vi "test Set Change on Parent.vi"(8 "error in":errorcluster, 11 "TestCase in":refnum<class "Refresh.lvclass">) -> (0 "error out":errorcluster, 3 "TestCase out":refnum<class "Refresh.lvclass">)   [LabVIEW 2020, in "Refresh.lvclass"]
uses:
  Refresh.lvclass
  System Explorer/Implementation/System Explorer/Refresh/MCL Row.ctl
  System Explorer/Implementation/System Explorer/Refresh/Change Type.ctl
  System Explorer/Implementation/System Explorer/Refresh/Symbols.ctl
  Scripting/Constants.vi
  <vilib>/addons/_JKI Toolkits/VI Tester/TestCase.llb/TestCase.lvclass
  System Explorer/Implementation/System Explorer/Refresh/Refresh.lvlib
  Scripting/AIM MIL-STD-1553 Scripting.lvlib
  C:/Program Files (x86)/National Instruments/LabVIEW 2020/vi.lib/addons/_JKI Toolkits/VI Tester/TestCase.llb/TestCase.lvclass
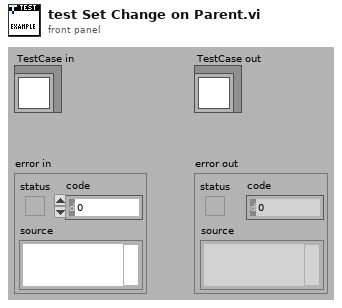
[diagram p1: front panel]
types:
  T1 = typedef "AIM MIL-STD-1553 System Explorer.lvlib/Implementation.lvlib/Refresh.lvlib/MCL Row.ctl" = cluster{"change type":T2, "item symbol":T3, "item names":string[]}
  T2 = typedef "AIM MIL-STD-1553 System Explorer.lvlib/Implementation.lvlib/Refresh.lvlib/Change Type.ctl" = enum16{"No change", "Modify", "Add", "Remove"}
  T3 = typedef "AIM MIL-STD-1553 System Explorer.lvlib/Implementation.lvlib/Refresh.lvlib/Symbols.ctl" = enum16{"Blank", "MIL-STD-1553", "Port", "Remote Terminal", "Subaddress", "Bus Controller", "Frame", "Mode Code", "Message", "Parameter", "Item"}
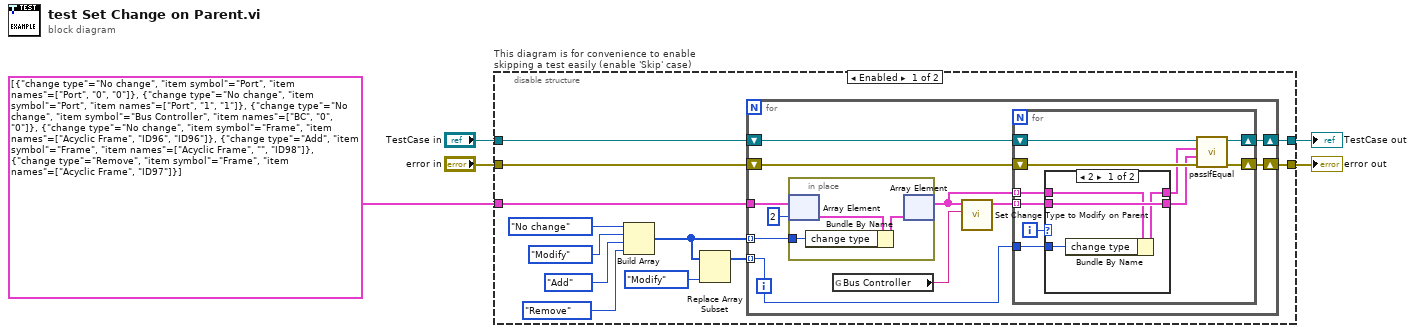
[diagram p0: block diagram]
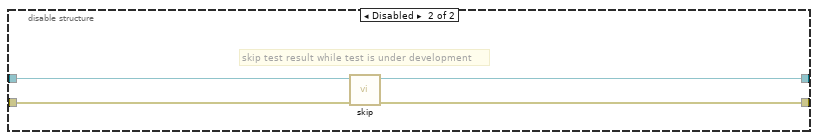
[diagram p3: hidden frame]
diagram:
  n1 = disable-structure "This diagram is for convenience to enable skipping a test easily (enable 'Skip' case)" shown="Enabled" {
    disable-tunnel: "TestCase in" -> [w17 w51]
    disable-tunnel: [w15 w49] -> w2
    disable-tunnel: [w14 w50] -> w4
    disable-tunnel: "error in" -> [w16 w48]
    disable-tunnel: T1[] [{"change type"=enum."No change", "item symbol"=enum."Port", "item names"=["Port", "0", "0"]}, {"change type"=enum."No change", "item symbol"=enum."Port", "item names"=["Port", "1", "1"]}, {"change type"=enum."No change", "item symbol"=enum."Bus Controller", "item names"=["BC", "0", "0"]}, {"change type"=enum."No change", "item symbol"=enum."Frame", "item names"=["Acyclic Frame", "ID96", "ID96"]}, {"change type"=enum."Add", "item symbol"=enum."Frame", "item names"=["Acyclic Frame", "", "ID98"]}, {"change type"=enum."Remove", "item symbol"=enum."Frame", "item names"=["Acyclic Frame", "ID97"]}] ("refresh items in") -> [w13 _]
    frame Enabled {
      n2 = Build Array(Change_Type."No change" ("change type"), Change_Type."Modify" ("change type"), Change_Type."Add" ("change type"), Change_Type."Remove" ("change type")) -> (w7:T2[])
      n3 = Replace Array Subset(array=w7, new element=Change_Type."Modify" ("change type")) -> (w6:T2[])  [unwired: 1 in]
      n4 = for {
        tunnel: w13 -> [w24]
        shift-right: [w26] -> w15
        shift-left: w17 -> [w28]
        shift-right: [w25] -> w14
        shift-left: w16 -> [w27]
        tunnel: w7 -> [w21] mode=indexing
        tunnel: w6 -> [w18] mode=indexing
        n5 = in-place {
          in-place-border: w21 -> [w29]
          n6 = in-place-array #1(w24, 2) -> (w31:T1)
          n7 = Bundle By Name(cluster=w31, "change type"=w29) -> (w30:T1)
          n8 = in-place-array #1(w30) -> (w19:T1[])  [unwired: 1 out]
        }
        n9 = global read "Constants.vi" "Bus Controller"() -> (w22:string)
        n10 = call "Set Change Type to Modify on Parent.vi"("parent name"=w22, "refresh items in"=w19) -> ("refresh items out"=w20:T1[])  [unwired: 9 in]
        n11 = for {
          shift-right: [w34] -> w26
          shift-left: w28 -> [w36]
          shift-right: [w35] -> w25
          shift-left: w27 -> [w37]
          tunnel: w20 -> [w40] mode=indexing
          tunnel: w19 -> [w41] mode=indexing
          tunnel: w18 -> [w38]
          i -> [w39]
          n12 = case shown="2" w39 {
            tunnel: w41 -> [w44 w47]
            tunnel: w40 -> [w45 w46]
            tunnel: w38 -> [w43 _]
            tunnel: [w42 w47] -> w33
            tunnel: [w45 w46] -> w32
            frame 2 {
              n13 = Bundle By Name(cluster=w44, "change type"=w43) -> (w42:T1)
            }
            frame Default {
            }
          }
          n14 = call-dynamic "passIfEqual.vi"("error in (no error)"=w37, "y"=w32, "x"=w33, "TestCase in"=w36) -> ("error out"=w35:errorcluster, "TestCase out"=w34:refnum<class "Refresh.lvclass">)  [unwired: 6 in]
        }
      }
    }
    frame Disabled {
      # "skip test result while test is under development"
      n15 = call <vilib>:"skip.vi"("error in (no error)"=w48, "TestCase in"=w51) -> ("error out"=w50:errorcluster, "TestCase out"=w49:refnum<class "Refresh.lvclass">)  [unwired: 8 in]
    }
  }
  "error out" <- w4
  "TestCase out" <- w2
